vi "save excel.vi"(0 "Path to Save Report":path=path "C:/excel files/1.xls", 1 "Enable":bool=TRUE, 2 "Additional_Comments":variant, 3 "Author_Name":variant, 4 "Comments":variant, 5 "Company_Name":variant, 6 "Graph1_Data_Input":variant, 7 "error in (no error)":errorcluster, 8 "Graph2_Data_Input":variant, 9 "Operator_Name":variant, 10 "Report_Title_Main":variant, 11 "Table1_Data_Input":variant, 12 "Table2_Data_Input":variant, 13 "Title1_Data_Input":variant, 14 "Title2_Data_Input":variant) -> (21 "Saved Report Path":path, 27 "error out":errorcluster)   [LabVIEW 2019]
doc: "Allows you to configure Word and Excel reports using templates. You can use basic templates that the LabVIEW Report Generation Toolkit for Microsoft Office includes, or you can create templates in Word and Excel.\n--------------------\n\nThis Express VI is configured as follows:\n\nTemplate Type: Basic Report for Excel\nDestination: Save to File"
uses:
  <vilib>/addons/_office/MSOfficeReportShared.llb/ex_RGT_Block State Information.ctl
  <vilib>/addons/_office/MSOfficeReportShared.llb/ex_RGT_Value Source.ctl
  <vilib>/addons/_office/MSOfficeReportShared.llb/ex_RGT_Input Appearance In Report.ctl
  <vilib>/addons/_office/MSOfficeReportShared.llb/ex_RGT_System Defined Value.ctl
  <vilib>/addons/_office/NI_ReportGenerationToolkit.lvlib
panel:
  in  "Bkm25":variant
  in  "Bkm24":variant
  in  "Bkm23":variant
  in  "Bkm22":variant
  in  "Bkm21":variant
  in  "Bkm20":variant
  in  "Template":u16(ring) items=["Basic Excel Template", "Basic Word Template", "Custom Excel Template", "Custom Word Template"]
  in  "Bkm19":variant
  in  "Bkm18":variant
  in  "Printer Settings":T1={"Printer Name"="", "Number of Copies"=1}
  in  "Bkm16":variant
  in  "Bkm13":variant
  in  "Bkm14":variant
  in  "Bkm15":variant
  in  "Bkm17":variant
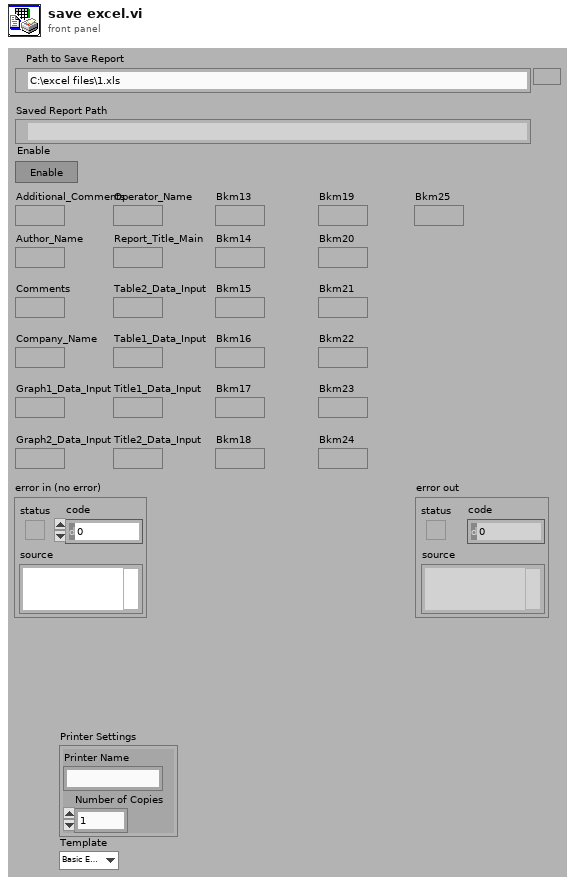
[diagram p1: front panel]
types:
  T1 = cluster{"Printer Name":string, "Number of Copies":i16}
  T2 = typedef "NI_ReportGenerationToolkit.lvlib/ex_RGT_Block State Information.ctl" = cluster{"Bookmark":string, "Value Source":T3, "Input Appearance in Report":T4, "Fixed Value":string, "System Defined Value":T5}
  T3 = typedef "NI_ReportGenerationToolkit.lvlib/ex_RGT_Value Source.ctl" = u16
  T4 = typedef "NI_ReportGenerationToolkit.lvlib/ex_RGT_Input Appearance In Report.ctl" = u16
  T5 = typedef "NI_ReportGenerationToolkit.lvlib/ex_RGT_System Defined Value.ctl" = u16
  T6 = enum16{"overwrite & backup", "next avail", "overwrite"}
  T7 = cluster{"HLP_Date Type":u16, "HLP_MDY":u16, "HLP_year":u16}
  T8 = cluster{"HLP_Time Type":u16, "HLP_Hour Type":u16, "HLP_HMS":u16}
  T9 = cluster{"format string for bookmark as Date":string, "format string for bookmark as Time":string}
  T10 = cluster{"BookMark/NamedCell":string, "Data":variant}
  T11 = cluster{"BookMark/NamedCell":string, "Data":variant}[]
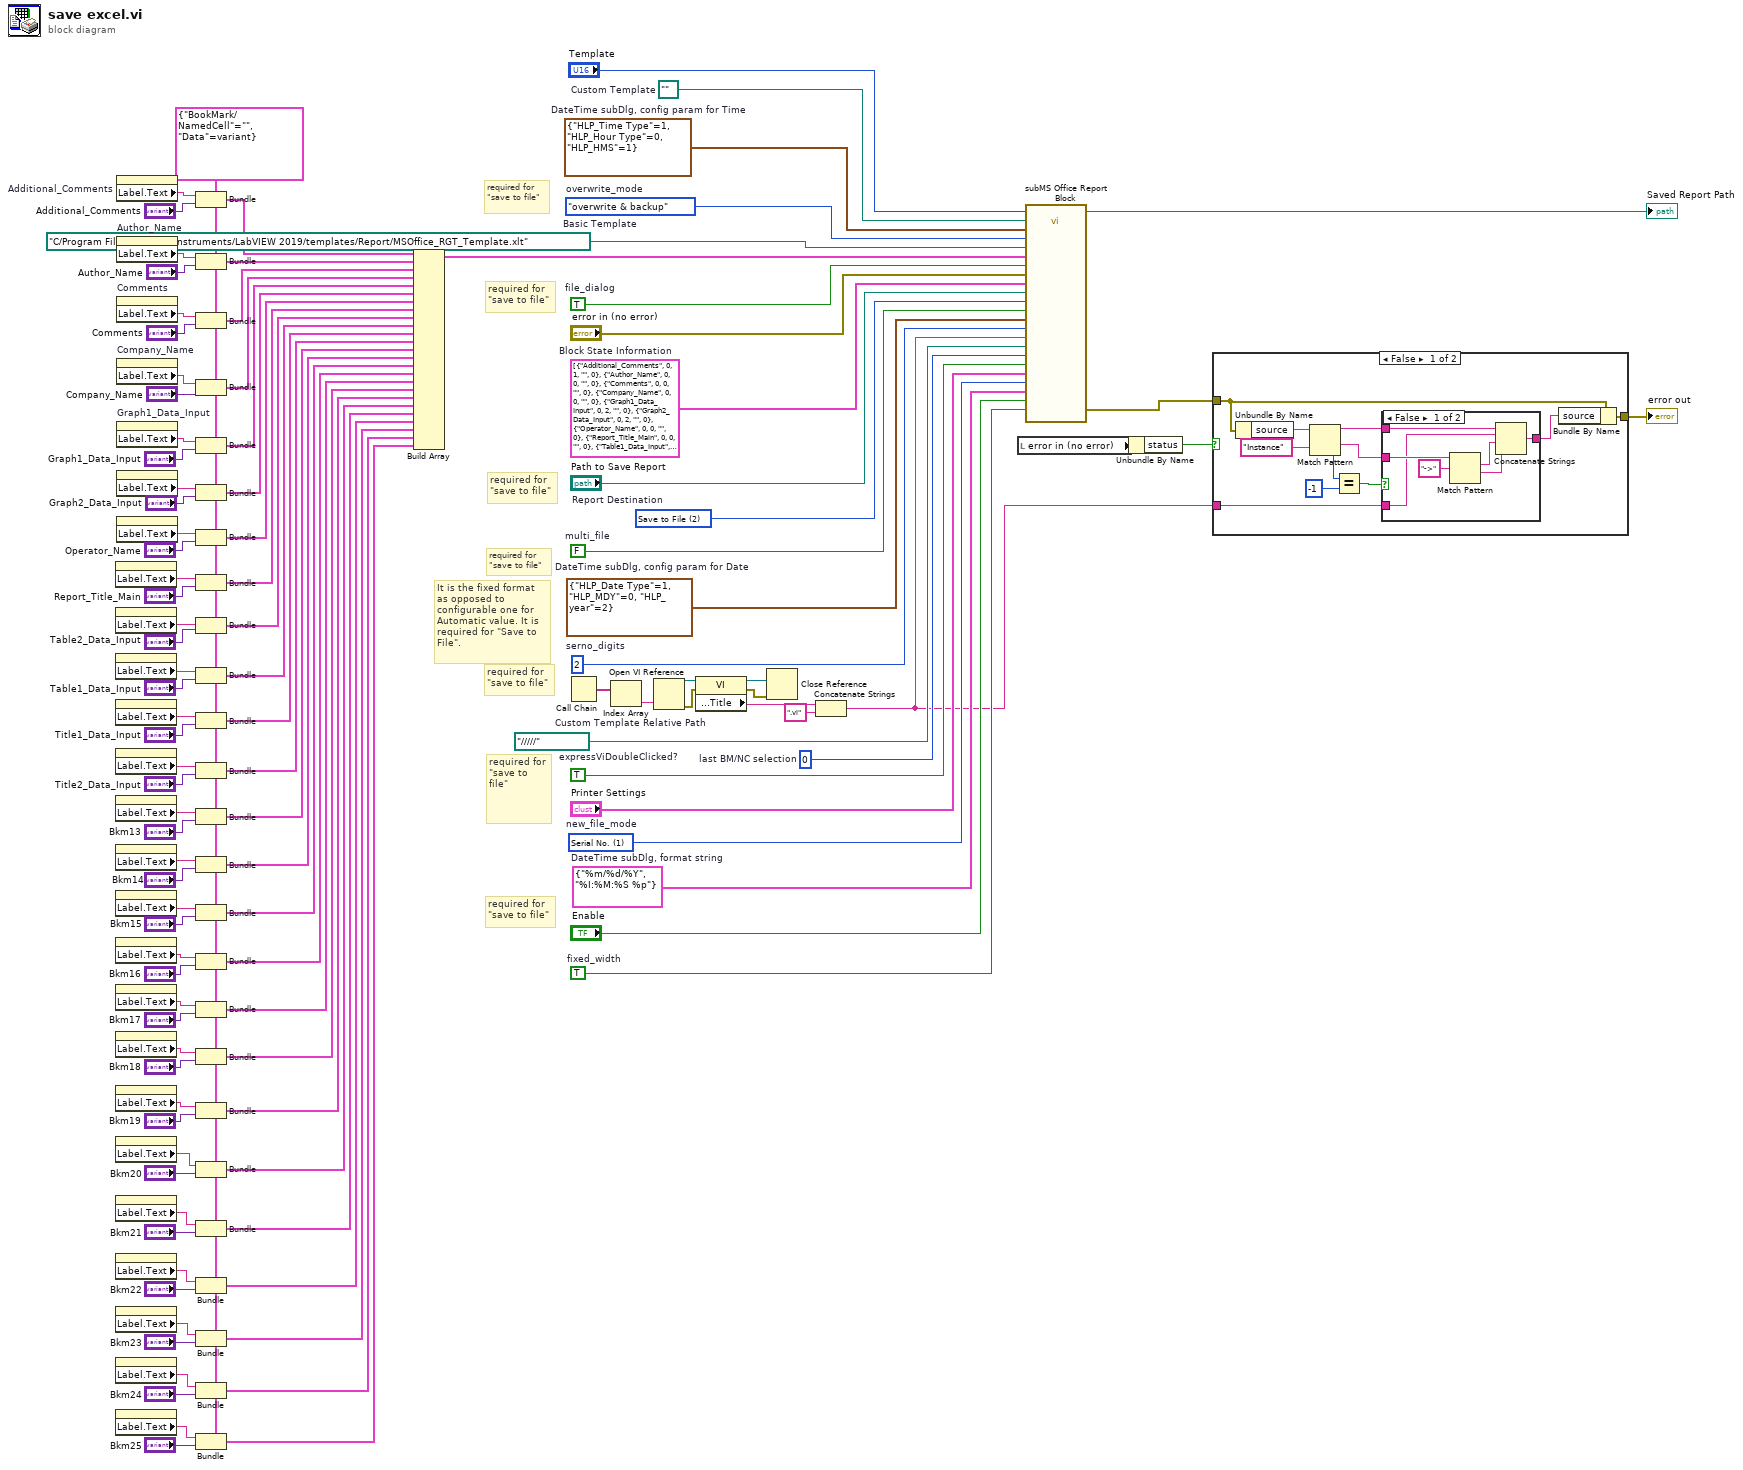
[diagram p0: block diagram]
diagram:
  w29 = path "../../../../../.."  # Custom Template Relative Path
  w37 = T2[] [{"Bookmark"="Additional_Comments", "Value Source"=0, "Input Appearance in Report"=1, "Fixed Value"="", "System Defined Value"=0}, {"Bookmark"="Author_Name", "Value Source"=0, "Input Appearance in Report"=0, "Fixed Value"="", "System Defined Value"=0}, {"Bookmark"="Comments", "Value Source"=0, "Input Appearance in Report"=0, "Fixed Value"="", "System Defined Value"=0}, {"Bookmark"="Company_Name", "Value Source"=0, "Input Appearance in Report"=0, "Fixed Value"="", "System Defined Value"=0}, {"Bookmark"="Graph1_Data_Input", "Value Source"=0, "Input Appearance in Report"=2, "Fixed Value"="", "System Defined Value"=0}, {"Bookmark"="Graph2_Data_Input", "Value Source"=0, "Input Appearance in Report"=2, "Fixed Value"="", "System Defined Value"=0}, {"Bookmark"="Operator_Name", "Value Source"=0, "Input Appearance in Report"=0, "Fixed Value"="", "System Defined Value"=0}, {"Bookmark"="Report_Title_Main", "Value Source"=0, "Input Appearance in Report"=0, "Fixed Value"="", "System Defined Value"=0}, {"Bookmark"="Table1_Data_Input", "Value Source"=0, "Input Appearance in Report"=0, "Fixed Value"="", "System Defined Value"=0}, {"Bookmark"="Table2_Data_Input", "Value Source"=0, "Input Appearance in Report"=0, "Fixed Value"="", "System Defined Value"=0}, {"Bookmark"="Title1_Data_Input", "Value Source"=0, "Input Appearance in Report"=0, "Fixed Value"="", "System Defined Value"=0}, {"Bookmark"="Title2_Data_Input", "Value Source"=0, "Input Appearance in Report"=0, "Fixed Value"="", "System Defined Value"=0}]  # Block State Information
  w40 = T6."overwrite & backup"  # overwrite_mode
  w41 = 0  # last BM/NC selection
  w42 = T7 {"HLP_Date Type"=1, "HLP_MDY"=0, "HLP_year"=2}  # DateTime subDlg, config param for Date
  w43 = T8 {"HLP_Time Type"=1, "HLP_Hour Type"=0, "HLP_HMS"=1}  # DateTime subDlg, config param for Time
  w45 = T9 {"format string for bookmark as Date"="%m/%d/%Y", "format string for bookmark as Time"="%I:%M:%S %p"}  # DateTime subDlg, format string
  w39 = u16 2 items=["Open in Microsoft Office", "Print to Printer", "Save to File"]  # Report Destination
  w38 = TRUE  # expressViDoubleClicked?
  w97 = path ""  # Custom Template
  w91 = u16 1 items=["Date & Time", "Serial No.", "Both"]  # new_file_mode
  w92 = TRUE  # fixed_width
  w93 = 2  # serno_digits
  w94 = FALSE  # multi_file
  w46 = TRUE  # file_dialog
  w6 = T10 {"BookMark/NamedCell"="", "Data"=variant} ("cluster")
  w96 = path "C:/Program Files/National Instruments/LabVIEW 2019/templates/Report/MSOffice_RGT_Template.xlt"  # Basic Template
  # "It is the fixed format as opposed to configurable one for Automatic value. It is required for \"Save to File\"."
  # "required for \n\"save to file\""
  # "required for \n\"save to file\""
  # "required for \n\"save to file\""
  # "required for \n\"save to file\""
  # "required for \n\"save to file\""
  # "required for \n\"save to file\""
  # "required for \n\"save to file\""
  n1 = property on="Report_Title_Main" class="LVVar"() -> ("Label.Text"=w86:string)  [unwired: 2 in, 2 out]
  n2 = property on="Table2_Data_Input" class="LVVar"() -> ("Label.Text"=w84:string)  [unwired: 2 in, 2 out]
  n3 = property on="Table1_Data_Input" class="LVVar"() -> ("Label.Text"=w82:string)  [unwired: 2 in, 2 out]
  n4 = property on="Title1_Data_Input" class="LVVar"() -> ("Label.Text"=w80:string)  [unwired: 2 in, 2 out]
  n5 = property on="Title2_Data_Input" class="LVVar"() -> ("Label.Text"=w78:string)  [unwired: 2 in, 2 out]
  n6 = property on="Bkm13" class="LVVar"() -> ("Label.Text"=w76:string)  [unwired: 2 in, 2 out]
  n7 = property on="Bkm14" class="LVVar"() -> ("Label.Text"=w74:string)  [unwired: 2 in, 2 out]
  n8 = property on="Bkm15" class="LVVar"() -> ("Label.Text"=w72:string)  [unwired: 2 in, 2 out]
  n9 = property on="Bkm16" class="LVVar"() -> ("Label.Text"=w70:string)  [unwired: 2 in, 2 out]
  n10 = property on="Bkm17" class="LVVar"() -> ("Label.Text"=w68:string)  [unwired: 2 in, 2 out]
  n11 = property on="Bkm18" class="LVVar"() -> ("Label.Text"=w52:string)  [unwired: 2 in, 2 out]
  n12 = property on="Bkm19" class="LVVar"() -> ("Label.Text"=w51:string)  [unwired: 2 in, 2 out]
  n13 = property on="Bkm20" class="LVVar"() -> ("Label.Text"=w18:string)  [unwired: 2 in, 2 out]
  n14 = property on="Bkm21" class="LVVar"() -> ("Label.Text"=w15:string)  [unwired: 2 in, 2 out]
  n15 = property on="Bkm22" class="LVVar"() -> ("Label.Text"=w13:string)  [unwired: 2 in, 2 out]
  n16 = property on="Bkm23" class="LVVar"() -> ("Label.Text"=w11:string)  [unwired: 2 in, 2 out]
  n17 = property on="Bkm24" class="LVVar"() -> ("Label.Text"=w9:string)  [unwired: 2 in, 2 out]
  n18 = property on="Bkm25" class="LVVar"() -> ("Label.Text"=w7:string)  [unwired: 2 in, 2 out]
  n19 = property on="Additional_Comments" class="LVVar"() -> ("Label.Text"=w112:string)  [unwired: 2 in, 2 out]
  n20 = property on="Author_Name" class="LVVar"() -> ("Label.Text"=w110:string)  [unwired: 2 in, 2 out]
  n21 = property on="Comments" class="LVVar"() -> ("Label.Text"=w108:string)  [unwired: 2 in, 2 out]
  n22 = property on="Company_Name" class="LVVar"() -> ("Label.Text"=w106:string)  [unwired: 2 in, 2 out]
  n23 = property on="Graph1_Data_Input" class="LVVar"() -> ("Label.Text"=w104:string)  [unwired: 2 in, 2 out]
  n24 = property on="Graph2_Data_Input" class="LVVar"() -> ("Label.Text"=w90:string)  [unwired: 2 in, 2 out]
  n25 = property on="Operator_Name" class="LVVar"() -> ("Label.Text"=w88:string)  [unwired: 2 in, 2 out]
  n26 = Bundle(cluster=w6, "BookMark/NamedCell"=w112, "Data"="Additional_Comments") -> (w102:T10)
  n27 = Bundle(cluster=w6, "BookMark/NamedCell"=w110, "Data"="Author_Name") -> (w101:T10)
  n28 = Bundle(cluster=w6, "BookMark/NamedCell"=w108, "Data"="Comments") -> (w100:T10)
  n29 = Bundle(cluster=w6, "BookMark/NamedCell"=w106, "Data"="Company_Name") -> (w99:T10)
  n30 = Bundle(cluster=w6, "BookMark/NamedCell"=w104, "Data"="Graph1_Data_Input") -> (w98:T10)
  n31 = Bundle(cluster=w6, "BookMark/NamedCell"=w90, "Data"="Graph2_Data_Input") -> (w66:T10)
  n32 = Bundle(cluster=w6, "BookMark/NamedCell"=w88, "Data"="Operator_Name") -> (w65:T10)
  n33 = Bundle(cluster=w6, "BookMark/NamedCell"=w86, "Data"="Report_Title_Main") -> (w64:T10)
  n34 = Bundle(cluster=w6, "BookMark/NamedCell"=w84, "Data"="Table2_Data_Input") -> (w63:T10)
  n35 = Bundle(cluster=w6, "BookMark/NamedCell"=w82, "Data"="Table1_Data_Input") -> (w62:T10)
  n36 = Bundle(cluster=w6, "BookMark/NamedCell"=w80, "Data"="Title1_Data_Input") -> (w61:T10)
  n37 = Bundle(cluster=w6, "BookMark/NamedCell"=w78, "Data"="Title2_Data_Input") -> (w60:T10)
  n38 = Bundle(cluster=w6, "BookMark/NamedCell"=w76, "Data"="Bkm13") -> (w59:T10)
  n39 = Bundle(cluster=w6, "BookMark/NamedCell"=w74, "Data"="Bkm14") -> (w58:T10)
  n40 = Bundle(cluster=w6, "BookMark/NamedCell"=w72, "Data"="Bkm15") -> (w57:T10)
  n41 = Bundle(cluster=w6, "BookMark/NamedCell"=w70, "Data"="Bkm16") -> (w56:T10)
  n42 = Bundle(cluster=w6, "BookMark/NamedCell"=w68, "Data"="Bkm17") -> (w55:T10)
  n43 = Bundle(cluster=w6, "BookMark/NamedCell"=w52, "Data"="Bkm18") -> (w49:T10)
  n44 = Bundle(cluster=w6, "BookMark/NamedCell"=w51, "Data"="Bkm19") -> (w48:T10)
  n45 = Bundle(cluster=w6, "BookMark/NamedCell"=w18, "Data"="Bkm20") -> (w17:T10)
  n46 = Bundle(cluster=w6, "BookMark/NamedCell"=w15, "Data"="Bkm21") -> (w5:T10)
  n47 = Bundle(cluster=w6, "BookMark/NamedCell"=w13, "Data"="Bkm22") -> (w4:T10)
  n48 = Bundle(cluster=w6, "BookMark/NamedCell"=w11, "Data"="Bkm23") -> (w3:T10)
  n49 = Bundle(cluster=w6, "BookMark/NamedCell"=w9, "Data"="Bkm24") -> (w2:T10)
  n50 = Bundle(cluster=w6, "BookMark/NamedCell"=w7, "Data"="Bkm25") -> (w1:T10)
  n51 = Build Array(w102, w101, w100, w99, w98, w66, w65, w64, w63, w62, w61, w60, w59, w58, w57, w56, w55, w49, w48, w17, w5, w4, w3, w2, w1) -> (w95:T11)
  n52 = Call Chain() -> (call chain=w28:string[])
  n53 = Index Array(array=w28) -> (element=w27:string)  [unwired: 1 in]
  n54 = Open VI Reference(vi path=w27) -> (vi reference=w26:refnum<vi>, error out=w25:errorcluster)  [unwired: 1 in, 4 out]
  n55 = property class="VI"(reference=w26, error in=w25) -> (reference out=w23:refnum<vi>, error out=w24:errorcluster, "Front Panel Window:Title"=w22:string)
  n56 = Close Reference(reference=w23, error in (no error)=w24) -> ()  [unwired: 1 out]
  n57 = Concatenate Strings(w22, ".vi" ("string")) -> (w20:string)
  n58 = local read "error in (no error)"() -> (w31:errorcluster)
  n59 = call <vilib>:"subMS Office Report Block.vi"("Template"="Template", "Custom Template"=w97, "DateTime subDlg, config param for Time"=w43, "overwrite_mode"=w40, "Basic Template"=w96, "Template Data"=w95, "file_dialog"=w46, "error in (no error)"="error in (no error)", "fixed_width"=w92, "Block State Information"=w37, "Enable"="Enable", "Path to Save Report"="Path to Save Report", "DateTime subDlg, format string"=w45, "Report Destination"=w39, "new_file_mode"=w91, "multi_file"=w94, "Printer Settings"="Printer Settings", "DateTime subDlg, config param for Date"=w42, "expressViDoubleClicked?"=w38, "serno_digits"=w93, "last BM/NC selection"=w41, "Custom Template Relative Path"=w29, "Block Label"=w20) -> ("Saved Report Path"=→"Saved Report Path":path, "error out"=w32:errorcluster)  [unwired: 3 out]
  n60 = Unbundle By Name(w31) -> ("status"=w30:bool)
  n61 = case shown="False" w30 {
    tunnel: [w114 w132] -> w33
    tunnel: w32 -> [w115 w132]
    tunnel: w20 -> [w113 _]
    frame False {
      n62 = Unbundle By Name(w115) -> ("source"=w123:string)
      n63 = Match Pattern(string=w123, regular expression="Instance") -> (before substring=w118:string, after substring=w117:string, offset past match=w120:i32)  [unwired: 2 out]
      n64 = Equal?(x=w120, y=-1) -> (x = y?=w121:bool)
      n65 = case shown="False" w121 {
        tunnel: [w125 w131] -> w116
        tunnel: w118 -> [w130 w131]
        tunnel: w117 -> [w128 _]
        tunnel: w113 -> [w124 _]
        frame False {
          n66 = Match Pattern(string=w128, regular expression="->") -> (match substring=w127:string, after substring=w126:string)  [unwired: 3 out]
          n67 = Concatenate Strings(w130, w124, w127, w126) -> (w125:string)
        }
        frame True {
        }
      }
      n68 = Bundle By Name(cluster=w115, "source"=w116) -> (w114:errorcluster)
    }
    frame True {
    }
  }
  "error out" <- w33
